vi "getCameraData.vi"(8 "error in (no error)":errorcluster, 10 "Array":u32[](array[numeric]), 11 "Refnum in":T1) -> (0 "error out":errorcluster, 2 "arrayOut":u32[](array[numeric]), 3 "Refnum out":T1)   [LabVIEW 2016]
uses:
  <vilib>/vision/Image Controls.llb/IMAQ Image.ctl
  Program Files (x86)/National Instruments/LabVIEW 2015/user.lib/cameraLibrary/cameraLibrary.lvlib
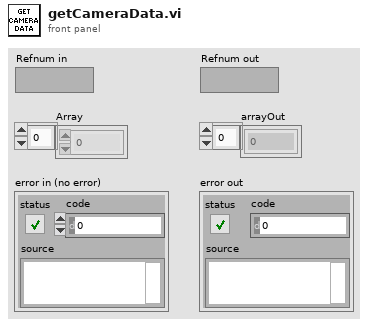
[diagram p1: front panel]
types:
  T1 = typedef "IMAQ Image.ctl" = refnum<image>
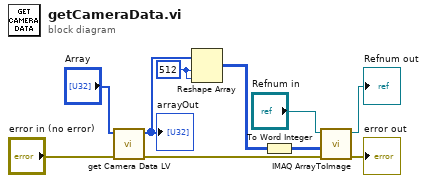
[diagram p0: block diagram]
diagram:
  w5 = 512
  n1 = call "get Camera Data LV.vi"("error in (no error)"="error in (no error)", "dataIn"="Array") -> ("error out"=w6:errorcluster, "dataOut"=w1:u32[])  [unwired: 8 in]
  "arrayOut" <- w1
  n2 = Reshape Array(w1, w5, w5) -> (w3:u32[][])
  n3 = To Word Integer(number=w3) -> (16bit integer=w2:i16[][])
  n4 = call "IMAQ ArrayToImage"("error in (no error)"=w6, "Image Pixels (I16)"=w2, "Image"="Refnum in") -> ("error out"=→"error out":errorcluster, "Image Out"=→"Refnum out":T1)  [unwired: 7 in]
